vi "acc and mag.vi"() -> ()   [LabVIEW 2021]
uses:
  <vilib>/Analysis/baseanly.llb/Mean (DBL).vi
  <vilib>/Utility/file.llb/Read Delimited Spreadsheet (I64).vi
  <vilib>/Analysis/NI_AALBase.lvlib
panel:
  in  "File path":path
  out "Magnitude vs Time":dbl[][](graph)
  out "subarray":i64[][](array[numeric])
  out "all rows":i64[][](array[numeric])
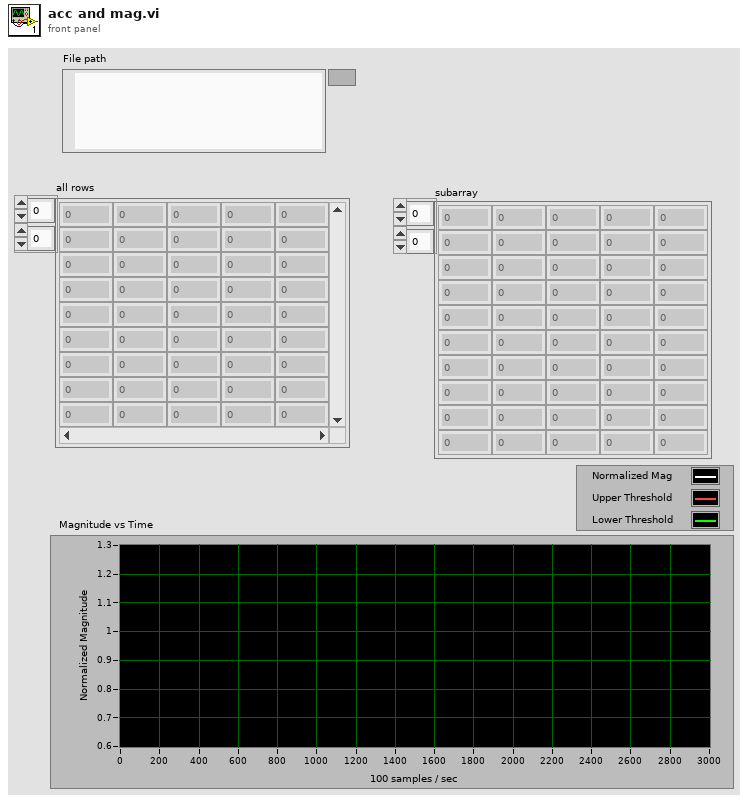
[diagram p1: front panel]
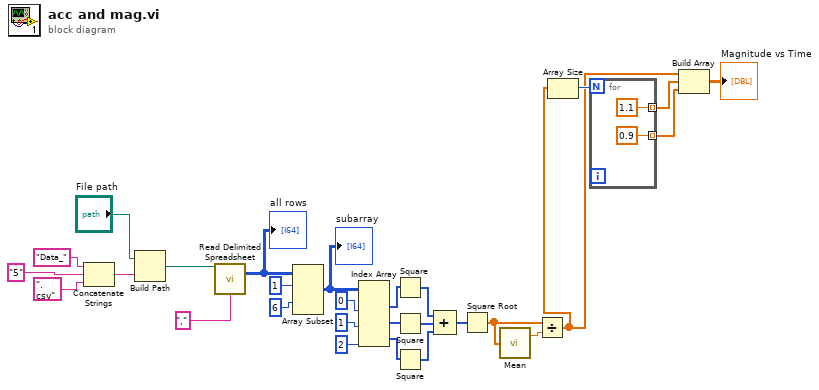
[diagram p0: block diagram]
diagram:
  n1 = Concatenate Strings("Data_" ("string"), "5" ("string"), ".csv" ("string")) -> (w12:string)
  n2 = Build Path(base path="File path", name or relative path=w12) -> (appended path=w24:path)
  n3 = call-poly <vilib>:"Read Delimited Spreadsheet.vi"("file path (dialog if empty)"=w24, "delimiter (\\t)"="," ("delimiter (\\t)")) -> ("all rows"=w23:i64[][])  [unwired: 8 in, 5 out]
  "all rows" <- w23
  n4 = Array Subset(array=w23, index (row)=1 ("index"), index (col)=6 ("index")) -> (w22:i64[][])  [unwired: 2 in]
  "subarray" <- w22
  n5 = Index Array(array=w22, index (col) #1=0 ("index (row)"), index (col) #2=1 ("index (row)"), index (col) #3=2 ("disabled index (col)")) -> (element #1=w21:i64[], element #2=w20:i64[], element #3=w19:i64[])  [unwired: 3 in]
  n6 = Square(x=w21) -> (x^2=w18:i64[])
  n7 = Square(x=w20) -> (x^2=w17:i64[])
  n8 = Square(x=w19) -> (x^2=w16:i64[])
  n9 = Compound Arithmetic op=ADD(w18, w17, w16) -> (w15:i64[])
  n10 = Square Root(x=w15) -> (sqrt(x)=w14:dbl[])
  n11 = call-poly <vilib>:"Mean.vi"("X"=w14) -> ("mean"=w13:dbl)  [unwired: 1 out]
  n12 = Divide(x=w14, y=w13) -> (x/y=w2:dbl[])
  n13 = Array Size(array=w2) -> (size(s)=w25:i32)
  n14 = for {
    N: w25 -> [_]
    tunnel: [0.9] -> w27 mode=indexing
    tunnel: [1.1] -> w26 mode=indexing
  }
  n15 = Build Array(w2, w26, w27) -> (→"Magnitude vs Time":dbl[][])
